vi "Step 5 - Generate Lowpass for FPGA (Lowpass).vi"() -> ()   [LabVIEW 2023]
doc: "Demonstrates how to use the DFD FXP Code Generator VI to generate LabVIEW field-programmable gate array (FPGA) code.\n\nComplete the following steps to use this VI.\n1) Set the <B>Destination Folder</B> that contains all the generated VIs and the LabVIEW project.\n2) Run the VI.\n3) The <B>Max Input Fs@40 MHz FPGA Clock</B> output returns a value that indicates the processing power of the generated filter block.\n\nWhen this VI finishes generating the LabVIEW FPGA code, this VI opens the generated LabVIEW project automatically."
uses:
  <vilib>/addons/Digital Filter Design/_Objects.llb/DFD Coef Norm Type.ctl
  <vilib>/addons/Digital Filter Design/FXPModel.llb/DFD FXP Quantize Coef (Easy).vi
  <vilib>/addons/Digital Filter Design/CodeGen.llb/DFD FXP LabVIEW FPGA Code Generator.vi
  <vilib>/addons/Digital Filter Design/NI_DigFilterLicensed.lvlib
panel:
  out "Maximum Input Fs@40 MHz FPGA Clock":dbl format="%#_5p Hz"
  in  "# Channels":i32=1
  in  "Filter Name":string="Lowpass"
  in  "Destination Folder":path
  # "Select Help>>Show Context Help and move the cursor over the VI icon for more information."
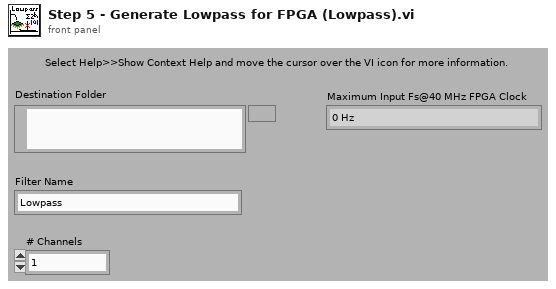
[diagram p1: front panel]
types:
  T1 = typedef "NI_DigFilterLicensed.lvlib/DFD Coef Norm Type.ctl" = enum16{"No Norm", "Time Domain 1-Norm", "Time Domain 2-Norm", "Time Domain Inf-Norm"}
  T2 = typedef "NI_DigFilterLicensed.lvlib/DFD Filter Obj.ctl" = cluster{"mSRate_Fs":dbl, "mSRate_Version":string, "mSRate_Comments":string, "mSRate_OrgCoef":T3, "mSRate_CurCoef":T3, "mSRate_Quantized?":bool, "mSRate_QCoef":T3, "mSRate_QSettings":T5[], "mSRate_Order":i32, "mSRate_Scaling":cluster{"mSRate_ScaleByPowerOf2?":bool, "mSRate_ScaleType":T1}}
  T3 = typedef "NI_DigFilterLicensed.lvlib/DFD Filter Coef.ctl" = cluster{"type":T4, "gain":dbl, "coef a (k)":dbl[], "coef b (v)":dbl[]}
  T4 = typedef "NI_DigFilterLicensed.lvlib/DFD Filter Structure Type Selector.ctl" = enum16{"Undefined", "FIR Direct Form", "FIR Direct Form Transposed", "FIR Symmetric", "FIR Antisymmetric", "IIR Direct Form I", "IIR Direct Form I Transposed", "IIR Direct Form II", "IIR Direct Form II Transposed", "IIR Cascaded Second Order Sections Form I", "IIR Cascaded Second Order Sections Form I Transposed", "IIR Cascaded Second Order Sections Form II", "IIR Cascaded Second Order Sections Form II Transposed", "Lattice Allpass (basic sections)", "Lattice Allpass (one multiplier sections)", "Lattice Allpass (normalized sections)", "Lattice AR (basic sections)", "Lattice AR (one multiplier sections)", "Lattice AR (normalized sections)", "Lattice MA (minimum phase)", "Lattice MA (maximum phase)", "Lattice ARMA (basic sections)", "Lattice ARMA (one multiplier sections)", "Lattice ARMA (normalized sections)"}
  T5 = typedef "NI_DigFilterLicensed.lvlib/dfd_Internal Quantization Settings.ctl" = cluster{"source":T6, "wl":i16, "iwl":i16, "overflow mode":enum16{"Saturation", "Wrap"}, "rounding mode":enum16{"Nearest", "Truncation"}, "signed?":bool}
  T6 = typedef "NI_DigFilterLicensed.lvlib/dfd_Internal Quantization Srcs.ctl" = u16
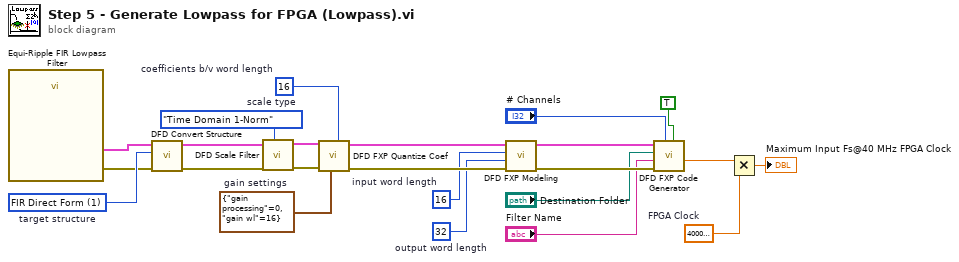
[diagram p0: block diagram]
diagram:
  w4 = i16 32  # output word length
  w3 = i16 16  # input word length
  w5 = i16 16  # coefficients b/v word length
  w6 = 40000000.0  # FPGA Clock
  w23 = u16 1 items=["FIR Direct Form"=1, "FIR Direct Form Transposed"=2, "FIR Symmetric"=3, "FIR Antisymmetric"=4, "IIR Direct Form I"=5, "IIR Direct Form I Transposed"=6, "IIR Direct Form II"=7, "IIR Direct Form II Transposed"=8, "IIR Cascaded Second-Order Sections Form I"=9, "IIR Cascaded Second-Order Sections Form I Transposed"=10, "IIR Cascaded Second-Order Sections Form II"=11, "IIR Cascaded Second-Order Sections Form II Transposed"=12, "Lattice Allpass (basic sections)"=13, "Lattice Allpass (one multiplier sections)"=14, "Lattice Allpass (normalized sections)"=15, "Lattice AR (basic sections)"=16, "Lattice AR (one multiplier sections)"=17, "Lattice AR (normalized sections)"=18, "Lattice MA (minimum phase)"=19, "Lattice MA (maximum phase)"=20, "Lattice ARMA (basic sections)"=21, "Lattice ARMA (one multiplier sections)"=22, "Lattice ARMA (normalized sections)"=23]  # target structure
  w10 = cluster{"gain processing":u16, "gain wl":i16} {"gain processing"=0, "gain wl"=16}  # gain settings
  w11 = DFD_Coef_Norm_Type."Time Domain 1-Norm"  # scale type
  n1 = call "Equi-Ripple FIR Lowpass Filter"() -> ("error out"=w1:errorcluster, "filter out"=w2:T2)  [unwired: 1 in, 9 out]
  n2 = call <vilib>:"DFD Convert Structure.vi"("error in (no error)"=w1, "target structure"=w23, "filter in"=w2) -> ("error out"=w17:errorcluster, "filter out"=w18:T2)  [unwired: 7 out]
  n3 = call <vilib>:"DFD Scale Filter.vi"("scale type"=w11, "error in (no error)"=w17, "filter in"=w18) -> ("error out"=w15:errorcluster, "filter out"=w16:T2)  [unwired: 7 out]
  n4 = call-poly <vilib>:"DFD FXP Quantize Coef.vi"("coefficients b/v word length"=w5, "gain settings"=w10, "error in (no error)"=w15, "filter in"=w16) -> ("error out"=w21:errorcluster, "filter out"=w22:T2)  [unwired: 1 in, 5 out]
  n5 = call <vilib>:"DFD FXP Modeling.vi"("error in (no error)"=w21, "output word length"=w4, "input word length"=w3, "filter in"=w22) -> ("error out"=w19:errorcluster, "filter out"=w20:T2)  [unwired: 3 in, 3 out]
  n6 = call-poly <vilib>:"DFD FXP Code Generator.vi"("open project? (F)"=TRUE, "# channels"="# Channels", "error in (no error)"=w19, "filter name"="Filter Name", "destination folder"="Destination Folder", "filter in"=w20) -> ("sampling frequency/FPGA clock"=w9:dbl)  [unwired: 1 in, 4 out]
  n7 = Multiply(x=w9, y=w6) -> (x*y=→"Maximum Input Fs@40 MHz FPGA Clock":dbl)
